vi "Clip-Ball_Api.vi"(6 "I2C Ref In":T1={"myRIO Reference"={"myRIO Model"=enum."Unknown", "myRIO Hardware Reference"={"Generic FPGA Reference"=refnum, "Allow multiple opens"=FALSE}}, "I2C Channels Enum"=enum."Not Connected", "I2C Configuration"={"I2C Transfer Rate"=enum."Fast mode (400 kbps)"}}, 8 "Error In":errorcluster, 11 "動作":enum16{"オ", "中", "右", "收回", "合併"}(ring)) -> (0 "Error Out":errorcluster)   [LabVIEW 2019]
uses:
  <vilib>/myRIO/Instrument Drivers/Onboard IO/I2C/typedefs/I2C Reference.ctl
  <vilib>/myRIO/Common/Instrument Driver Framework/Utilities/typedefs/myRIO Generic Hardware Reference.ctl
  <vilib>/myRIO/Common/Instrument Driver Framework/Utilities/typedefs/Hardware Version Enum.ctl
  <vilib>/myRIO/Common/Instrument Driver Framework/Utilities/typedefs/myRIO v1.0 Reference.ctl
  <vilib>/myRIO/Common/Instrument Driver Framework/Utilities/typedefs/Generic FPGA Reference.ctl
  <vilib>/myRIO/Common/Instrument Driver Framework/myRIO v1.0/I2C/typedefs/I2C Channels Enum.ctl
  <vilib>/myRIO/Instrument Drivers/Onboard IO/I2C/typedefs/I2C Configuration.ctl
  <vilib>/myRIO/Instrument Drivers/Onboard IO/I2C/typedefs/I2C Transfer Rate.ctl
  <vilib>/myRIO/Instrument Drivers/Onboard IO/I2C/I2C.lvlib
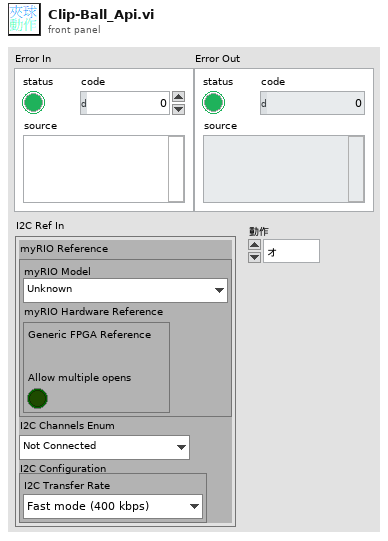
[diagram p1: front panel]
types:
  T1 = typedef "I2C.lvlib/I2C Reference.ctl" = cluster{"myRIO Reference":T2, "I2C Channels Enum":T6, "I2C Configuration":T7}
  T2 = typedef "myRIO Generic Hardware Reference.ctl" = cluster{"myRIO Model":T3, "myRIO Hardware Reference":T4}
  T3 = typedef "Hardware Version Enum.ctl" = enum16{"Unknown", "myRIO-1900", "myRIO-1950", "roboRIO", "NI ELVIS RIO CM", "ELVIS III"}
  T4 = typedef "myRIO v1.0 Reference.ctl" = cluster{"Generic FPGA Reference":T5, "Allow multiple opens":bool}
  T5 = typedef "Generic FPGA Reference.ctl" = refnum<k20>
  T6 = typedef "I2C Channels Enum.ctl" = enum16{"Not Connected", "A/I2C", "B/I2C", "I2C/I2C"}
  T7 = typedef "I2C.lvlib/I2C Configuration.ctl" = cluster{"I2C Transfer Rate":T8}
  T8 = typedef "I2C.lvlib/I2C Transfer Rate.ctl" = enum16{"Standard mode (100 kbps)", "Fast mode (400 kbps)"}
  T9 = enum16{"前", "後", "オ", "右", "無", "0", "1", "2", "3", "4", "5", "6", "7"}
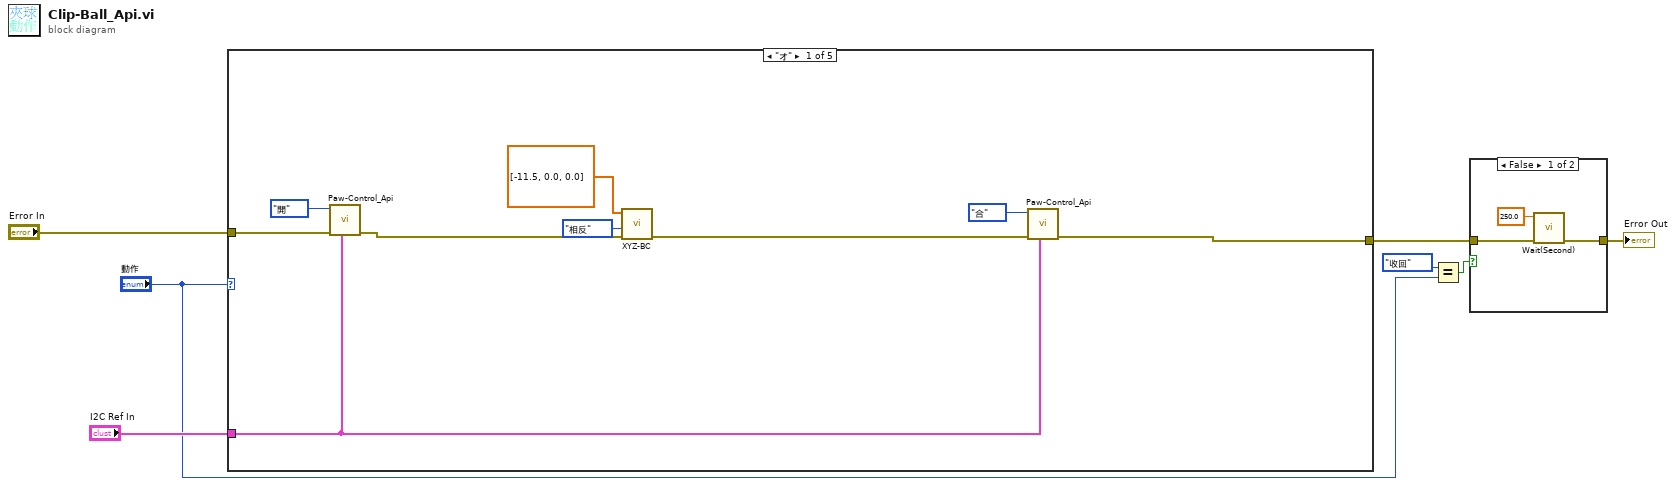
[diagram p0: block diagram]
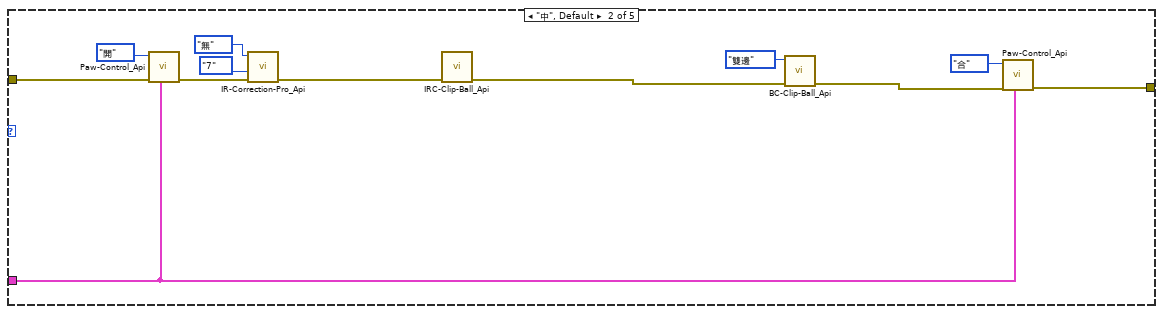
[diagram p3: hidden frame]
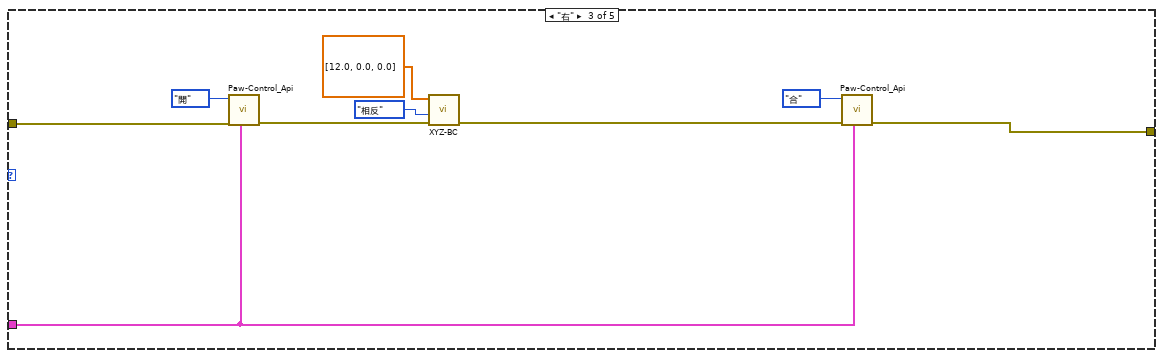
[diagram p4: hidden frame]
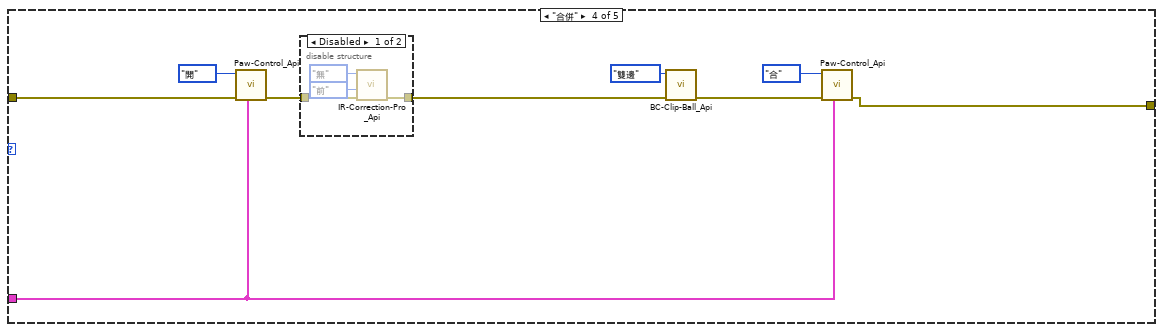
[diagram p5: hidden frame]
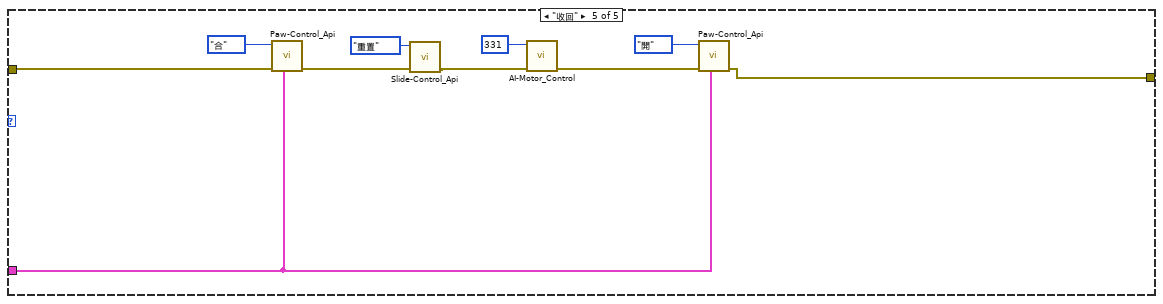
[diagram p7: hidden frame]
diagram:
  n1 = case shown="\"オ\"" "動作" {
    tunnel: "Error In" -> [w9 w21 w30 w41 w53]
    tunnel: [w14 w25 w35 w39 w56] -> w5
    tunnel: "I2C Ref In" -> [w13 w23 w34 w38 w54]
    frame "オ" {
      n2 = call "Paw-Control_Api.vi"("I2C Ref In"=w13, "Error In"=w9, "夾爪動作"=enum16{"開", "合"}."開") -> ("error out"=w8:errorcluster)  [unwired: 8 in]
      n3 = call "XYZ-BC.vi"("Error In"=w8, "校正微動位置"=enum16{"雙邊", "オ", "右", "相反"}."相反", "X-Y-Z移動"=dbl[] [-11.5, 0.0, 0.0]) -> ("Error Out"=w11:errorcluster)  [unwired: 8 in]
      n4 = call "Paw-Control_Api.vi"("I2C Ref In"=w13, "Error In"=w11, "夾爪動作"=enum16{"開", "合"}."合") -> ("error out"=w14:errorcluster)  [unwired: 8 in]
    }
    frame "中", Default {
      n5 = call "Paw-Control_Api.vi"("I2C Ref In"=w23, "Error In"=w21, "夾爪動作"=enum16{"開", "合"}."開") -> ("error out"=w22:errorcluster)  [unwired: 8 in]
      n6 = call "IR-Correction-Pro_Api.vi"("Error In"=w22, "副邊校正"=T9."7", "主編校正"=enum16{"前", "後", "オ", "右", "無"}."無") -> ("Error Out"=w18:errorcluster)  [unwired: 8 in]
      n7 = call "IRC-Clip-Ball_Api.vi"("Error In"=w18) -> ("Error Out"=w17:errorcluster)  [unwired: 10 in]
      n8 = call "BC-Clip-Ball_Api.vi"("Error In"=w17, "校正微動位置"=enum16{"雙邊", "オ", "右"}."雙邊") -> ("Error Out"=w19:errorcluster)  [unwired: 9 in]
      n9 = call "Paw-Control_Api.vi"("I2C Ref In"=w23, "Error In"=w19, "夾爪動作"=enum16{"開", "合"}."合") -> ("error out"=w25:errorcluster)  [unwired: 8 in]
    }
    frame "右" {
      n10 = call "Paw-Control_Api.vi"("I2C Ref In"=w34, "Error In"=w30, "夾爪動作"=enum16{"開", "合"}."開") -> ("error out"=w29:errorcluster)  [unwired: 8 in]
      n11 = call "XYZ-BC.vi"("Error In"=w29, "校正微動位置"=enum16{"雙邊", "オ", "右", "相反"}."相反", "X-Y-Z移動"=dbl[] [12.0, 0.0, 0.0]) -> ("Error Out"=w32:errorcluster)  [unwired: 8 in]
      n12 = call "Paw-Control_Api.vi"("I2C Ref In"=w34, "Error In"=w32, "夾爪動作"=enum16{"開", "合"}."合") -> ("error out"=w35:errorcluster)  [unwired: 8 in]
    }
    frame "合併" {
      n13 = call "Paw-Control_Api.vi"("I2C Ref In"=w38, "Error In"=w41, "夾爪動作"=enum16{"開", "合"}."開") -> ("error out"=w42:errorcluster)  [unwired: 8 in]
      n14 = disable-structure shown="Disabled" {
        disable-tunnel: w42 -> [w50 w51]
        disable-tunnel: [w47 w51] -> w40
        frame Disabled {
          n15 = call "IR-Correction-Pro_Api.vi"("Error In"=w50, "副邊校正"=T9."前", "主編校正"=enum16{"前", "後", "オ", "右", "無"}."無") -> ("Error Out"=w47:errorcluster)  [unwired: 8 in]
        }
        frame Enabled {
        }
      }
      n16 = call "BC-Clip-Ball_Api.vi"("Error In"=w40, "校正微動位置"=enum16{"雙邊", "オ", "右"}."雙邊") -> ("Error Out"=w43:errorcluster)  [unwired: 9 in]
      n17 = call "Paw-Control_Api.vi"("I2C Ref In"=w38, "Error In"=w43, "夾爪動作"=enum16{"開", "合"}."合") -> ("error out"=w39:errorcluster)  [unwired: 8 in]
    }
    frame "收回" {
      n18 = call "Paw-Control_Api.vi"("I2C Ref In"=w54, "Error In"=w53, "夾爪動作"=enum16{"開", "合"}."合") -> ("error out"=w52:errorcluster)  [unwired: 8 in]
      n19 = call "Slide-Control_Api.vi"("Error In"=w52, "狀態選擇"=enum16{"重置", "下降"}."重置") -> ("Error Out"=w58:errorcluster)  [unwired: 9 in]
      n20 = call "AI-Motor_Control.vi"("Error In"=w58, "目標位置(0~4095)"=u16 331) -> ("Error Out"=w60:errorcluster)  [unwired: 9 in]
      n21 = call "Paw-Control_Api.vi"("I2C Ref In"=w54, "Error In"=w60, "夾爪動作"=enum16{"開", "合"}."開") -> ("error out"=w56:errorcluster)  [unwired: 8 in]
    }
  }
  n22 = Equal?(x=enum16{"オ", "中", "右", "收回", "合併"}."收回", y="動作") -> (x = y?=w3:bool)
  n23 = case shown="False" w3 {
    tunnel: w5 -> [w64 w65]
    tunnel: [w63 w65] -> w4
    frame False {
      n24 = call "Wait(Second).vi"("Error In"=w64, "等待秒數(3000毫秒)"=250.0) -> ("Error Out"=w63:errorcluster)  [unwired: 9 in]
    }
    frame True {
    }
  }
  "Error Out" <- w4
